vi "Write gains.vi"(8 "error in (no error)":errorcluster, 10 "PI gains":T1 {"proportional gain" step=0.125}, 11 "BuckBoost configuration in":refnum<class "BuckBoost configuration.lvclass">) -> (0 "error out":errorcluster, 3 "BuckBoost configuration out":refnum<class "BuckBoost configuration.lvclass">)   [LabVIEW 2017, in "BuckBoost configuration.lvclass"]
uses:
  BuckBoost configuration.lvclass
  <vilib>/rvi/Analysis/control/PID/Typedef/niFpgaPID_PIGains.ctl
  BuckBoost configuration.lvclass/BuckBoost configuration.ctl
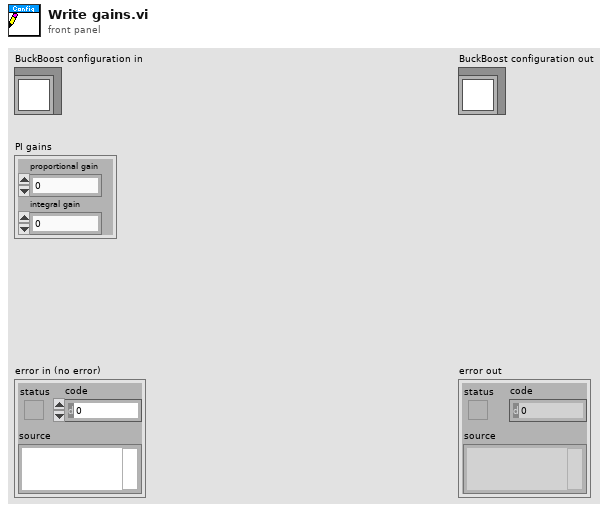
[diagram p1: front panel]
types:
  T1 = typedef "niFpgaPID_PIGains.ctl" = cluster{"proportional gain":sgl, "integral gain":sgl}
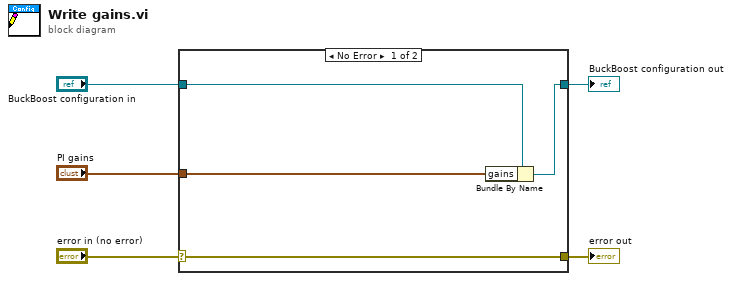
[diagram p0: block diagram]
diagram:
  n1 = case shown="No Error" "error in (no error)" {
    selector: "error in (no error)" -> [w9 w10]
    tunnel: [w9 w10] -> w4
    tunnel: [w7 w11] -> w2
    tunnel: "BuckBoost configuration in" -> [w8 w11]
    tunnel: "PI gains" -> [w6 _]
    frame No Error {
      n2 = Bundle By Name(cluster=w8, "gains"=w6) -> (w7:refnum<class "BuckBoost configuration.lvclass">)
    }
    frame Error {
    }
  }
  "error out" <- w4
  "BuckBoost configuration out" <- w2
